vi "New Entity Path.vi"(8 "Container Paths":path[](array[path]), 9 "Target":refnum<vi>, 10 "Entity Name":string, 11 "Container Index":i32) -> (3 "Default Entity Folder":path)   [LabVIEW 2020, in "Conditum-Tools.lvlib" / "Entity Editor.lvclass"]
uses:
  Entity Editor.lvclass
  Entity Editor.lvclass/Entity Editor.ctl
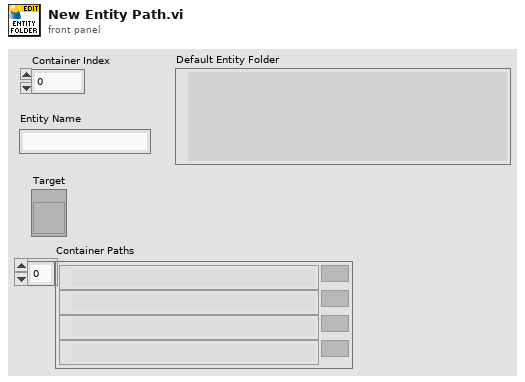
[diagram p1: front panel]
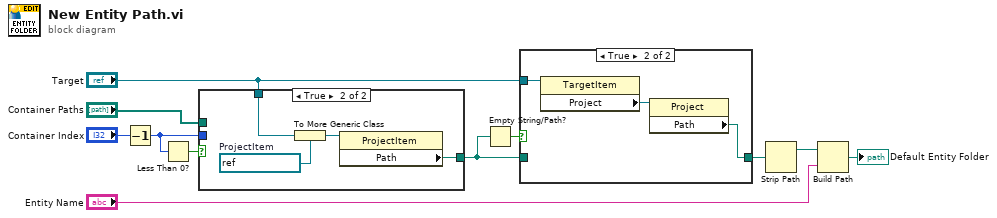
[diagram p0: block diagram]
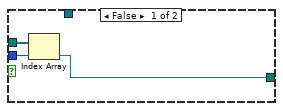
[diagram p2: hidden frame]
diagram:
  n1 = Decrement(x="Container Index") -> (x-1=w10:i32)
  n2 = Less Than 0?(x=w10) -> (x < 0?=w11:bool)
  n3 = case shown="True" w11 {
    tunnel: w10 -> [w13 _]
    tunnel: "Container Paths" -> [w14 _]
    tunnel: "Target" -> [_ w18]
    tunnel: [w12 w15] -> w1
    frame False {
      n4 = Index Array(array=w14, index=w13) -> (element=w12:path)
    }
    frame True {
      w17 = refnum<vi> refnum  # ProjectItem
      n5 = To More Generic Class(target class=w17, reference=w18) -> (generic class reference=w16:refnum<vi>)
      n6 = property class="ProjectItem"(reference=w16) -> ("Path"=w15:path)  [unwired: 1 in, 2 out]
    }
  }
  n7 = Empty String/Path?(string/path=w1) -> (empty?=w9:bool)
  n8 = case shown="True" w9 {
    tunnel: w1 -> [w19 _]
    tunnel: "Target" -> [_ w22]
    tunnel: [w19 w20] -> w6
    frame False {
    }
    frame True {
      n9 = property class="TargetItem"(reference=w22) -> ("Project"=w21:refnum<vi>)  [unwired: 1 in, 2 out]
      n10 = property class="Project"(reference=w21) -> ("Path"=w20:path)  [unwired: 1 in, 2 out]
    }
  }
  n11 = Strip Path(path=w6) -> (stripped path=w5:path)  [unwired: 1 out]
  n12 = Build Path(base path=w5, name or relative path="Entity Name") -> (appended path=→"Default Entity Folder":path)
